vi "3.2.0 Kalman State FG.vi"(2 "Covariance P 2":T1, 3 "State Variable X 2":T1, 4 "Enum":enum16{"get state", "set state"}(ring)) -> (0 "Covariance P":T1, 1 "State Variable X":T1)   [LabVIEW 2010]
uses:
  <vilib>/Analysis/Matrix/Datatypes/RealMatrix.ctl
  <vilib>/Analysis/Matrix/NI_Matrix.lvlib
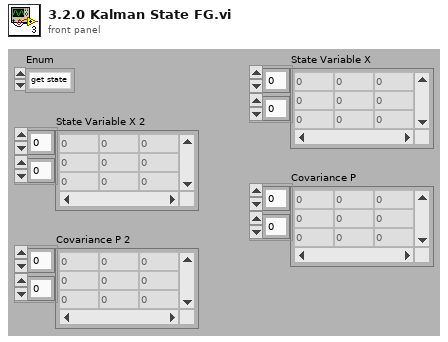
[diagram p1: front panel]
types:
  T1 = typedef "NI_Matrix.lvlib/RealMatrix.ctl" = dbl[][]
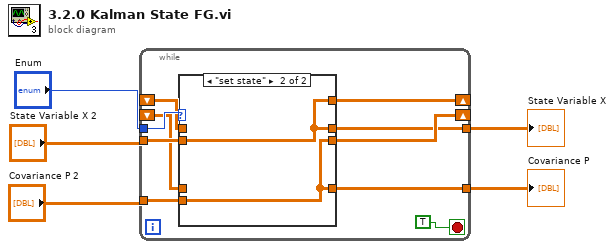
[diagram p0: block diagram]
diagram:
  n1 = while {
    shift-right: [w13] -> _
    shift-left: _ -> [w8]
    shift-right: [w11] -> _
    shift-left: _ -> [w6]
    tunnel: "Enum" -> [w14]
    tunnel: "State Variable X 2" -> [w12]
    tunnel: "Covariance P 2" -> [w10]
    tunnel: [w9] -> w4
    tunnel: [w7] -> w5
    stop <- TRUE stop-if-true
    n2 = case shown="\"set state\"" w14 {
      tunnel: [w17 w19] -> w13
      tunnel: w12 -> [_ w19]
      tunnel: [w16 w18] -> w11
      tunnel: w10 -> [_ w18]
      tunnel: [w17 w19] -> w9
      tunnel: w8 -> [w17 _]
      tunnel: [w16 w18] -> w7
      tunnel: w6 -> [w16 _]
      frame "get state", Default {
      }
      frame "set state" {
      }
    }
  }
  "Covariance P" <- w5
  "State Variable X" <- w4
